vi "runAmic.vi"() -> ()   [LabVIEW 2012]
uses:
  <vilib>/Utility/file.llb/Read From Spreadsheet File (string).vi
  <vilib>/addons/database/Connection.llb/DB Tools Open Connec (Path).vi
  <vilib>/addons/database/NI_Database_API.lvlib
panel:
  out "element 2":string
  out "error out 2":errorcluster
  out "error out 4":errorcluster
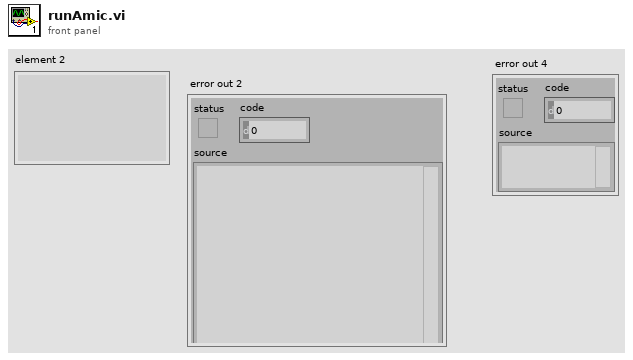
[diagram p1: front panel]
types:
  T1 = typedef "NI_Database_API.lvlib/Conn ObjectReference.ctl" = refnum<k1>
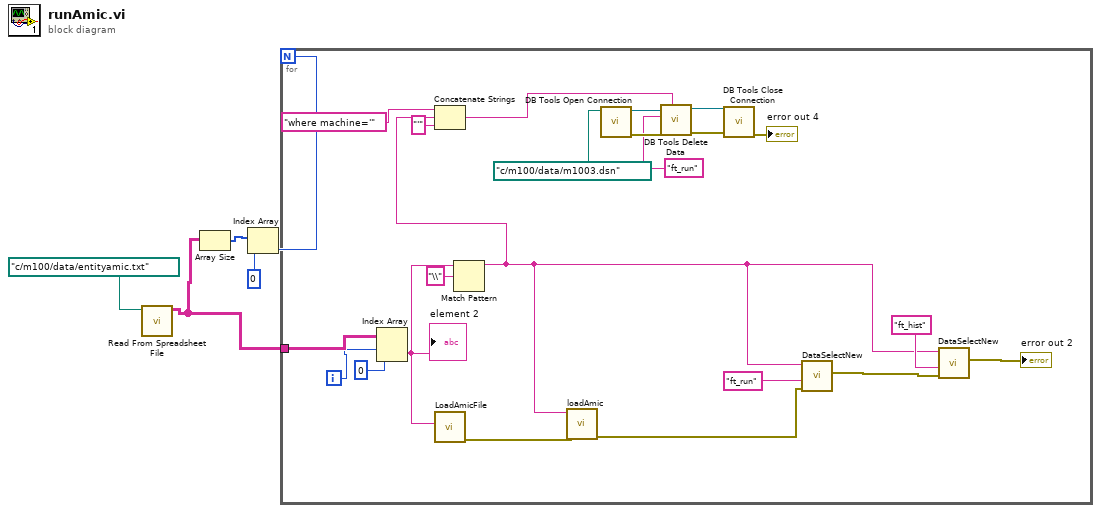
[diagram p0: block diagram]
diagram:
  n1 = call-poly <vilib>:"Read From Spreadsheet File.vi"("file path (dialog if empty)"=path "c:/m100/data/entityamic.txt" ("file path (use dialog)")) -> ("all rows"=w1:string[][])  [unwired: 6 in, 4 out]
  n2 = Array Size(array=w1) -> (size(s)=w4:i32[])
  n3 = Index Array(array=w4, index=0) -> (element=w2:i32)
  n4 = for {
    N: w2 -> [_]
    tunnel: w1 -> [w27]
    i -> [w25]
    n5 = Index Array(array=w27, index (row)=w25, index (col)=0 ("disabled index (col)")) -> (element=w9:string)
    "element 2" <- w9
    n6 = call "LoadAmicFile.vi"("folder"=w9) -> ("error out"=w8:errorcluster)  [unwired: 9 in, 1 out]
    n7 = Match Pattern(string=w9, regular expression="\\") -> (before substring=w6:string)  [unwired: 1 in, 3 out]
    n8 = Concatenate Strings("where machine='" ("string"), w6, "'" ("string")) -> (w10:string)
    n9 = call "loadAmic.vi"("error in"=w8, "machine"=w6) -> ("error out"=w7:errorcluster)  [unwired: 9 in]
    n10 = call-poly <vilib>:"DB Tools Open Connection.vi"("connection information"=path "c:/m100/data/m1003.dsn") -> ("error out"=w16:errorcluster, "connection reference"=w18:T1)  [unwired: 7 in]
    n11 = call <vilib>:"DB Tools Delete Data.vi"("condition"=w10, "error in (no error)"=w16, "table"="ft_run", "connection reference"=w18) -> ("error out"=w15:errorcluster, "connection reference out"=w17:T1)  [unwired: 6 in]
    n12 = call <vilib>:"DB Tools Close Connection.vi"("error in (no error)"=w15, "connection reference"=w17) -> ("error out"=→"error out 4":errorcluster)  [unwired: 5 in]
    n13 = call "DataSelectNew.vi"("error in (no error)"=w7, "Table"="ft_run", "Machine"=w6) -> ("error out"=w22:errorcluster)  [unwired: 8 in]
    n14 = call "DataSelectNew.vi"("error in (no error)"=w22, "Table"="ft_hist", "Machine"=w6) -> ("error out"=→"error out 2":errorcluster)  [unwired: 8 in]
  }
